vi "Send Notifier.vi"(8 "error in (no error)":errorcluster, 9 "Data":variant, 11 "Notifier In":refnum<queue>) -> (0 "error out":errorcluster)   [LabVIEW 2014]
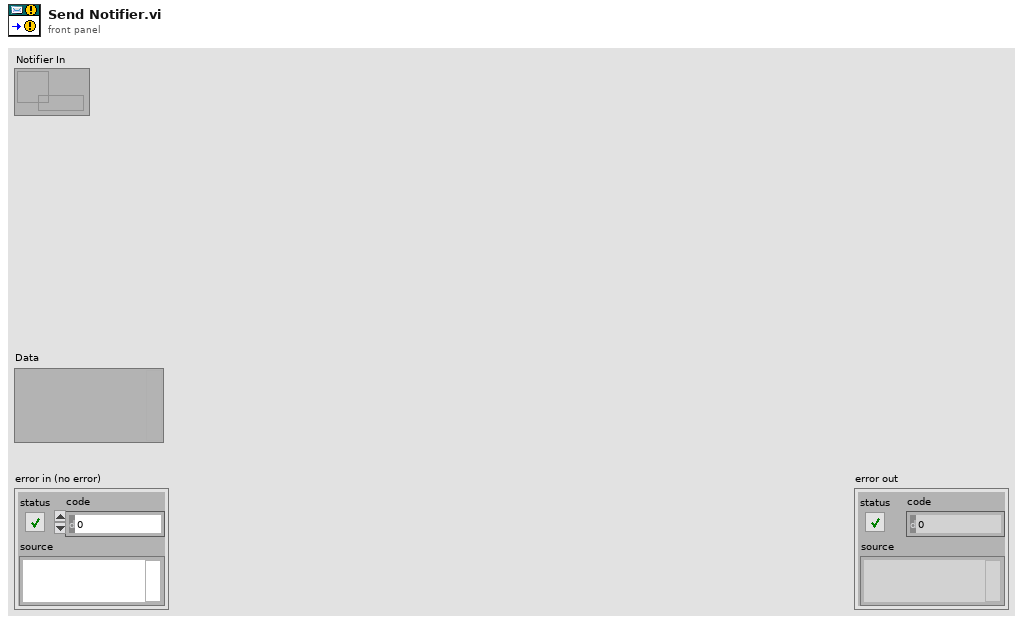
[diagram p1: front panel]
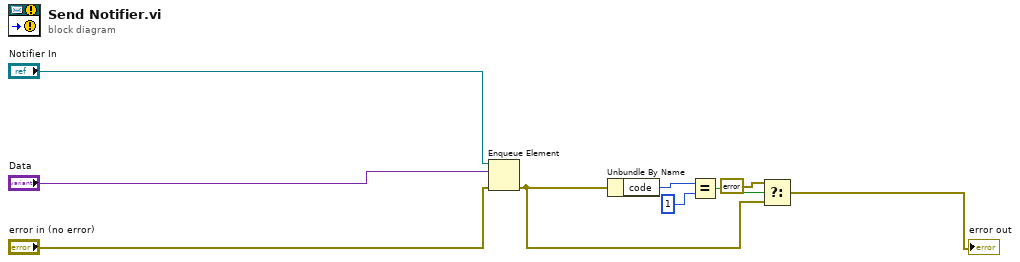
[diagram p0: block diagram]
diagram:
  n1 = Enqueue Element(queue="Notifier In", element="Data", error in (no error)="error in (no error)") -> (error out=w5:errorcluster)  [unwired: 1 in, 2 out]
  n2 = Unbundle By Name(w5) -> ("code"=w6:i32)
  n3 = Equal?(x=w6, y=1) -> (x = y?=w7:bool)
  n4 = Select(t=errorcluster {"status"=FALSE, "code"=0, "source"=""} ("error constant"), s=w7, f=w5) -> (s? t:f=→"error out":errorcluster)
